vi "Text file end.vi"(8 "error in":errorcluster, 11 "refnum file":refnum<file>) -> (0 "error out":errorcluster, 3 "refnum out":refnum<file>)   [LabVIEW 2013]
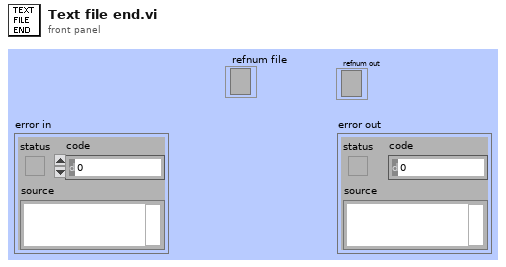
[diagram p1: front panel]
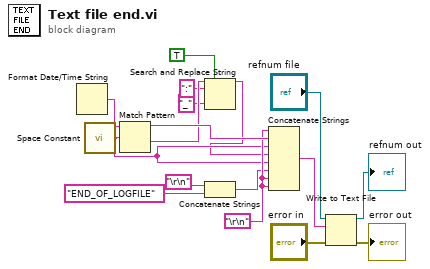
[diagram p0: block diagram]
diagram:
  w12 = "\r\n"
  n1 = Format Date/Time String() -> (date/time string=w16:string)  [unwired: 3 out]
  n2 = call <vilib>:"Space Constant.vi"() -> ("String"=w9:string)
  n3 = Match Pattern(string=w16, regular expression=w9) -> (before substring=w17:string, after substring=w5:string)  [unwired: 3 out]
  n4 = Search and Replace String(replace all?=TRUE ("replace all? (F)"), input string=w5, search string=":", replace string="_" ("replace string (\"\")")) -> (result string=w4:string)  [unwired: 1 in, 6 out]
  n5 = Concatenate Strings("\r\n", "END_OF_LOGFILE" ("string")) -> (w8:string)
  n6 = Concatenate Strings(w12, w17, w9, w4, w9, w8, w12, w12) -> (w15:string)
  n7 = Write to Text File(file (use dialog)="refnum file", text=w15, error in="error in") -> (refnum out=→"refnum out":refnum<file>, error out=→"error out":errorcluster)  [unwired: 2 out]
